vi "VI Name Wrapper.vi"(8 "error in (no error)":errorcluster, 11 "VI in":refnum<vi>) -> (0 "error out":errorcluster, 3 "Name":string)   [LabVIEW 2017, in "Promise Future.lvlib" / "Future.lvclass"]
uses:
  Future.lvclass
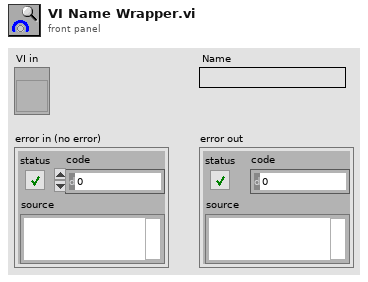
[diagram p1: front panel]
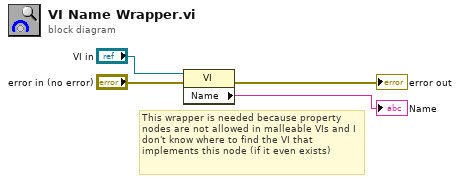
[diagram p0: block diagram]
diagram:
  # "This wrapper is needed because property nodes are not allowed in malleable VIs and I don't know where to find the VI that implements this node (if it even exists)"
  n1 = property class="VI"(reference="VI in", error in="error in (no error)") -> (error out=→"error out":errorcluster, "Name"=→"Name":string)  [unwired: 1 out]
